vi "NativeToStringPath.vi"(1 "Native Path":path) -> (0 "Agnostic Path":string)   [LabVIEW 2020]
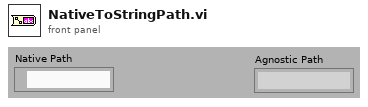
[diagram p1: front panel]
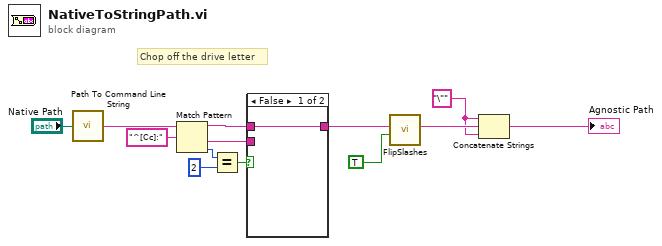
[diagram p0: block diagram]
diagram:
  w9 = "\"" ("string")
  # "Chop off the drive letter"
  n1 = call <vilib>:"Path To Command Line String.vi"("path"="Native Path") -> ("string"=w8:string)
  n2 = Match Pattern(string=w8, regular expression="^[Cc]:") -> (before substring=w4:string, after substring=w3:string, offset past match=w2:i32)  [unwired: 2 out]
  n3 = Equal?(x=w2, y=2) -> (x = y?=w5:bool)
  n4 = case shown="False" w5 {
    tunnel: w4 -> [w14 _]
    tunnel: w3 -> [_ w15]
    tunnel: [w14 w15] -> w7
    frame False {
    }
    frame True {
    }
  }
  n5 = call <vilib>:"FlipSlashes.vi"("ConfigFormat"=TRUE, "Before"=w7) -> ("After"=w11:string)  [unwired: 9 out]
  n6 = Concatenate Strings(w9, w11, w9) -> (→"Agnostic Path":string)
